vi "Get Logic Status.vi"   [LabVIEW 2016, in "Hardware.lvlib" / "LogicIO.lvlib" / "LogicIO.lvclass"]
uses:
  <userlib>/Common Components/Hardware/LogicIO/LogicIO/LogicIO.lvclass
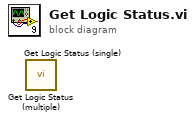
[diagram p0: block diagram]
diagram:
  n1 = call <userlib>:"Get Logic Status (multiple).vi"() -> ()  [unwired: 9 in, 3 out]
  n2 = call <userlib>:"Get Logic Status (single).vi"() -> ()  [unwired: 9 in, 3 out]
